vi "SV Refnum to Control.vi"(8 "error in (no error)":errorcluster, 11 "shared variable refnum in":refnum<k21>) -> (0 "error out":errorcluster, 3 "Shared Variable Control Out":refnum<k21>)   [LabVIEW 2026, in "TALOS.lvlib"]
doc: "Use this VI to convert a SV Refnum (used in the Programmatic Access) to a SV Control, used in the DS Module VIs."
uses:
  TALOS.lvlib
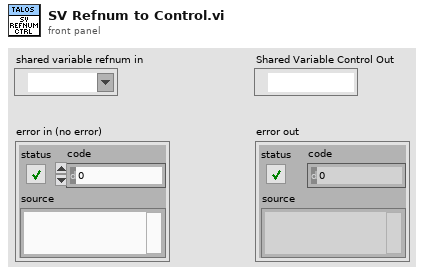
[diagram p1: front panel]
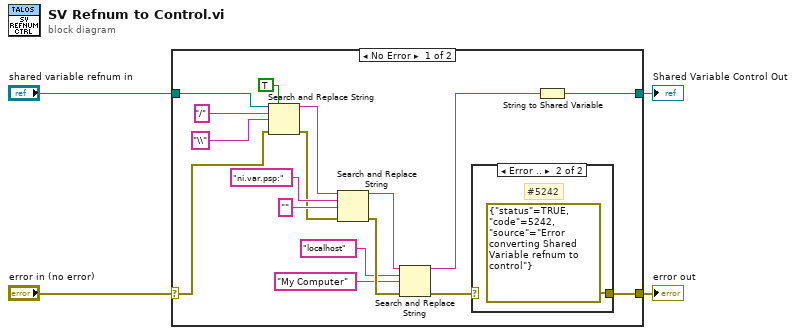
[diagram p0: block diagram]
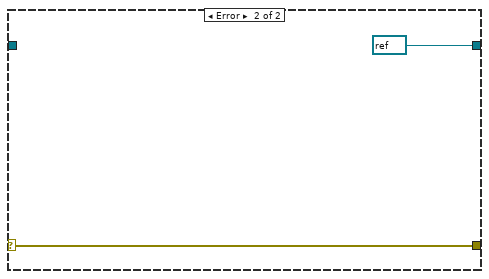
[diagram p3: hidden frame]
diagram:
  n1 = case shown="No Error" "error in (no error)" {
    selector: "error in (no error)" -> [w9 w25]
    tunnel: [w7 refnum<k21> refnum] -> w1
    tunnel: "shared variable refnum in" -> [w10 _]
    tunnel: [w5 w25] -> w3
    frame No Error {
      n2 = Search and Replace String(replace all?=TRUE ("replace all? (F)"), input string=w10, search string="/", replace string="\\" ("replace string (\"\")"), error in=w9) -> (result string=w18:string, error out=w15:errorcluster)  [unwired: 3 in, 2 out]
      n3 = Search and Replace String(input string=w18, search string="ni.var.psp:", replace string="" ("replace string (\"\")"), error in=w15) -> (result string=w13:string, error out=w14:errorcluster)  [unwired: 4 in, 2 out]
      n4 = Search and Replace String(input string=w13, search string="localhost", replace string="My Computer" ("replace string (\"\")"), error in=w14) -> (result string=w8:string, error out=w6:errorcluster)  [unwired: 4 in, 2 out]
      n5 = case shown="Error .." w6 {
        selector: w6 -> [w22 _]
        tunnel: [w22 errorcluster {"status"=TRUE, "code"=5242, "source"="Error converting Shared Variable refnum to control"} ("error IO")] -> w5
        frame No Error {
        }
        frame Error {
          # "#5242"
        }
      }
      n6 = String to Shared Variable(0:w8) -> (2:w7:refnum<k21>)  [unwired: 1 out]
    }
    frame Error {
    }
  }
  "error out" <- w3
  "Shared Variable Control Out" <- w1
